vi "Read Image In.vi"(8 "error in (no error)":errorcluster, 11 "HIJ Vision Display in":refnum<class "HIJ Vision Display.lvclass">) -> (0 "error out":errorcluster, 2 "Image":T1, 3 "HIJ Vision Display out":refnum<class "HIJ Vision Display.lvclass">)   [LabVIEW 2014, in "HIJ Vision Display.lvlib" / "HIJ Vision Display.lvclass"]
uses:
  HIJ Vision Display.lvclass
  <vilib>/vision/Image Controls.llb/IMAQ Image.ctl
  HIJ Vision Display.lvclass/HIJ Vision Display.ctl
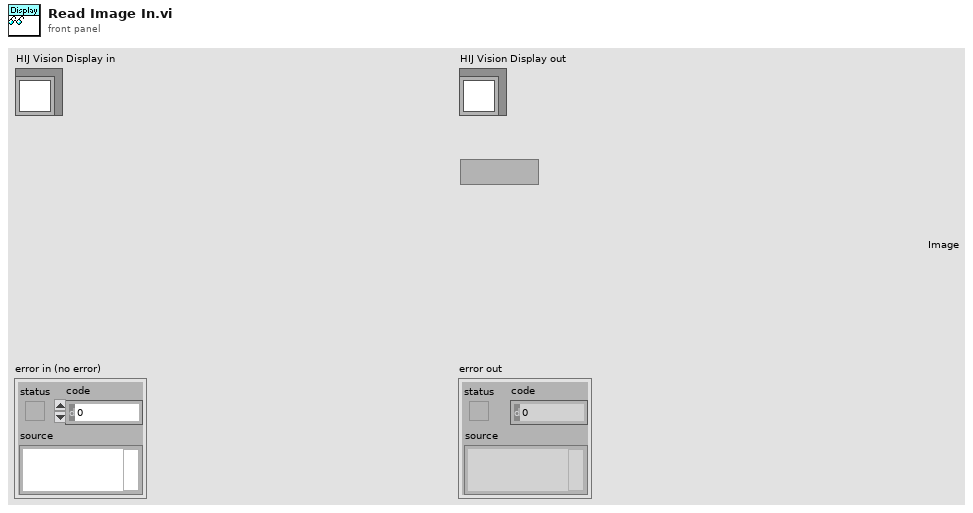
[diagram p1: front panel]
types:
  T1 = typedef "IMAQ Image.ctl" = refnum<image>
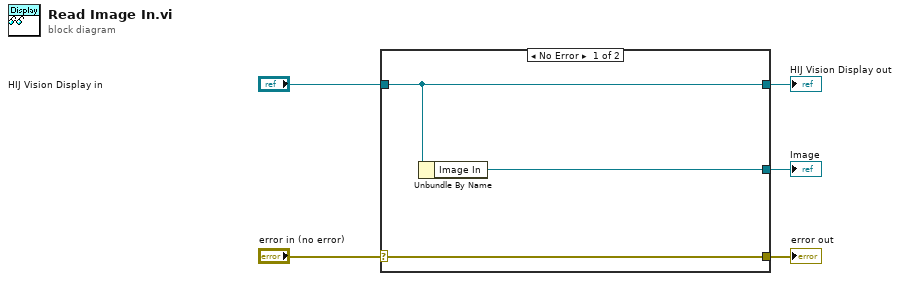
[diagram p0: block diagram]
diagram:
  n1 = case shown="No Error" "error in (no error)" {
    selector: "error in (no error)" -> [w8 w9]
    tunnel: [w8 w9] -> w4
    tunnel: [w7 w10] -> w2
    tunnel: "HIJ Vision Display in" -> [w7 w10]
    tunnel: [w6 _] -> w1
    frame No Error {
      n2 = Unbundle By Name(w7) -> ("Image In"=w6:T1)
    }
    frame Error {
    }
  }
  "error out" <- w4
  "HIJ Vision Display out" <- w2
  "Image" <- w1
